vi "Has Clients.vi"(8 "error in (no error)":errorcluster, 11 "Basic WebSocket Manager in":refnum<class "Basic WebSocket Manager.lvclass">) -> (0 "error out":errorcluster, 2 "Has Client(s)":bool, 3 "Basic WebSocket Manager out":refnum<class "Basic WebSocket Manager.lvclass">)   [LabVIEW 2020, in "HTTP Server.lvlib" / "Basic WebSocket Manager.lvclass"]
uses:
  Basic WebSocket Manager.lvclass
  Basic WebSocket Manager.lvclass/Basic WebSocket Manager.ctl
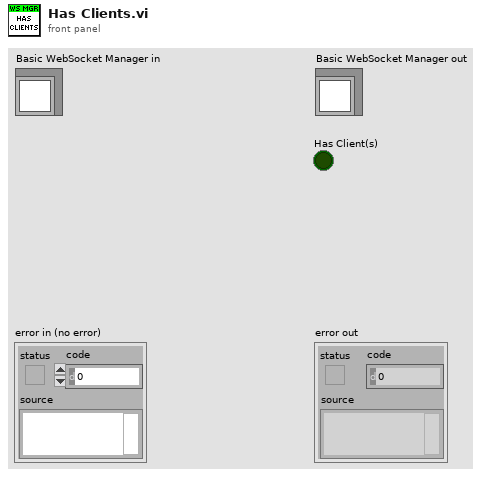
[diagram p1: front panel]
types:
  T1 = typedef "HTTP Server.lvlib/Basic WebSocket Manager.lvclass/Ref Data.ctl" = cluster{"Clients":map{string, refnum<class "WebSocket Client.lvclass">}}
  T2 = map{string, refnum<class "WebSocket Client.lvclass">}
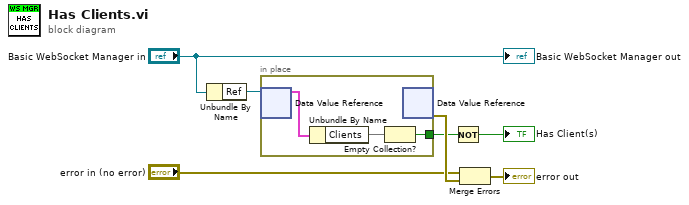
[diagram p0: block diagram]
diagram:
  n1 = Unbundle By Name("Basic WebSocket Manager in") -> ("Ref"=w5:refnum<data-value>)
  n2 = in-place {
    in-place-border: [w8] -> w3
    n3 = in-place-dvr #1(w5) -> (w10:T1)  [unwired: 1 out]
    n4 = Unbundle By Name(w10) -> ("Clients"=w9:T2)
    n5 = Empty Collection?(1:w9) -> (0:w8:bool)
    n6 = in-place-dvr #1() -> (w7:errorcluster)  [unwired: 1 in, 1 out]
  }
  n7 = Not(x=w3) -> (.not. x?=→"Has Client(s)":bool)
  n8 = Merge Errors("error in (no error)", w7) -> (→"error out":errorcluster)
  "Basic WebSocket Manager out" <- "Basic WebSocket Manager in"
